vi "strip illegal filename chars.vi"(11 "string in":string) -> (3 "string out":string)   [LabVIEW 2015]
panel:
  in  "illegal filename characters":string="/?<>\\:*|\"^\n"
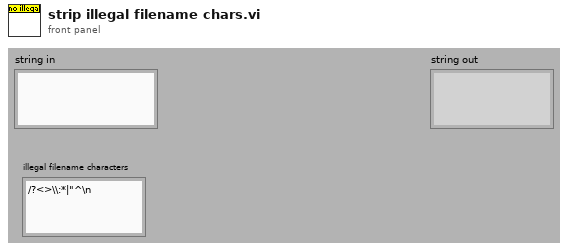
[diagram p1: front panel]
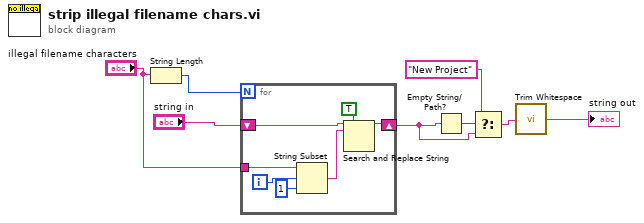
[diagram p0: block diagram]
diagram:
  n1 = String Length(string="illegal filename characters") -> (length=w8:i32)
  n2 = for {
    N: w8 -> [_]
    tunnel: "illegal filename characters" -> [w14]
    shift-right: [w9] -> w3
    shift-left: "string in" -> [w10]
    i -> [w13]
    n3 = String Subset(string=w14, offset (0)=w13, length (rest)=1 ("length (rest)")) -> (substring=w11:string)
    n4 = Search and Replace String(replace all?=TRUE ("replace all? (F)"), input string=w10, search string=w11) -> (result string=w9:string)  [unwired: 5 in, 3 out]
  }
  n5 = Empty String/Path?(string/path=w3) -> (empty?=w5:bool)
  n6 = Select(t="New Project", s=w5, f=w3) -> (s? t:f=w2:string)
  n7 = call <vilib>:"Trim Whitespace.vi"("string"=w2) -> ("trimmed string"=→"string out":string)  [unwired: 1 in]
